vi "Disconnect.vi"(8 "error in (no error)":errorcluster, 11 "SV B-M (Target) in":refnum<class "SV B-M (Target).lvclass">) -> (0 "error out":errorcluster, 3 "SV B-M (Target) out":refnum<class "SV B-M (Target).lvclass">)   [LabVIEW 2015, in "SV B-M (Target).lvclass"]
uses:
  SV B-M (Target).lvclass
  Command & Ack - Destroy Endpoints.vi
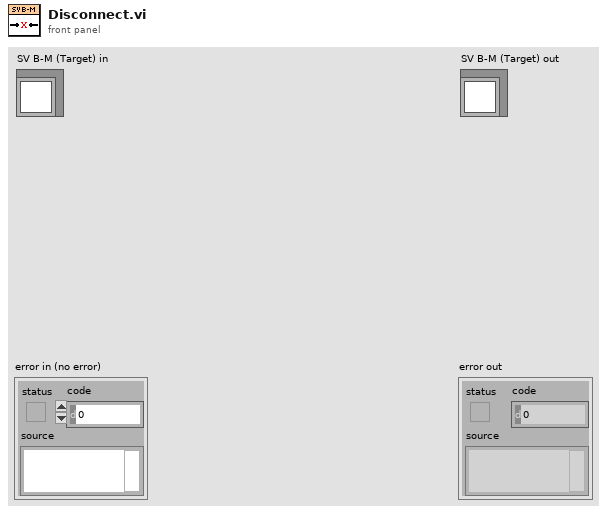
[diagram p1: front panel]
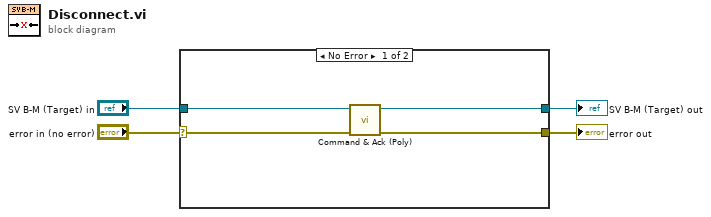
[diagram p0: block diagram]
diagram:
  n1 = case shown="No Error" "error in (no error)" {
    selector: "error in (no error)" -> [w7 w10]
    tunnel: [w5 w10] -> w3
    tunnel: [w6 w9] -> w1
    tunnel: "SV B-M (Target) in" -> [w8 w9]
    frame No Error {
      n2 = call-poly "Command & Ack (Poly).vi"("error in (no error)"=w7, "SV B-M (Target) in"=w8) -> ("error out"=w5:errorcluster, "SV B-M (Target) out"=w6:refnum<class "SV B-M (Target).lvclass">)  [unwired: 8 in]
    }
    frame Error {
    }
  }
  "error out" <- w3
  "SV B-M (Target) out" <- w1
